vi "RSZVB Calibration Kit Catalog With Label.vi"(8 "error in (no error)":errorcluster {"code" format="%.0x"}, 10 "Connector Name (\"\")":string, 11 "VISA session":refnum<visa-resource-name>) -> (0 "error out":errorcluster {"code" format="%.0x"}, 2 "Catalog":string, 3 "dup VISA session":refnum<visa-resource-name>)   [LabVIEW 2011]
doc: "This VI Returns a list of all cal kits and their labels for a given connector type.\n\nRemote-control command(s):\n[SENSe<Ch>:]CORRection:CKIT:LCATalog? '<Conn_Name>'"
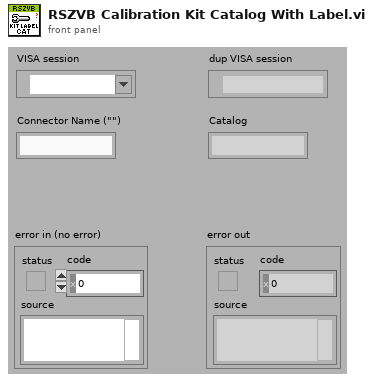
[diagram p1: front panel]
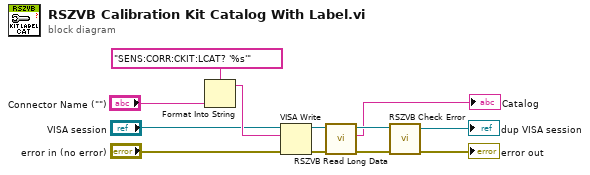
[diagram p0: block diagram]
diagram:
  n1 = Format Into String(format string="SENS:CORR:CKIT:LCAT? '%s'", "Connector Name (\"\")") -> (resulting string=w11:string)  [unwired: 2 in, 1 out]
  n2 = VISA Write(VISA resource name="VISA session", write buffer=w11, error in (no error)="error in (no error)") -> (VISA resource name out=w10:refnum<visa-resource-name>, error out=w9:errorcluster)  [unwired: 1 out]
  n3 = call "RSZVB Read Long Data.vi"("error in (no error)"=w9, "VISA resource name"=w10) -> ("error out"=w7:errorcluster, "Data"=→"Catalog":string, "VISA resource name out"=w8:refnum<visa-resource-name>)  [unwired: 7 in]
  n4 = call "RSZVB Check Error.vi"("error in (no error)"=w7, "VISA session"=w8) -> ("error out"=→"error out":errorcluster, "dup VISA session"=→"dup VISA session":refnum<visa-resource-name>)  [unwired: 8 in]
